vi "ActuationTransform_v6.vi"(8 "1/Actuation Radius":fxp<+,18,0>, 9 "U_thY":fxp<+/-,35,11>, 10 "U_thX":fxp<+/-,35,11>, 11 "U_z":fxp<+/-,35,11>) -> (1 "F_B (Left,B)":fxp<+/-,25,3> format="%.10f", 2 "F_G (Right, G)":fxp<+/-,25,3> format="%.10f", 3 "F_R (Top,R)":fxp<+/-,25,3> format="%.10f")   [LabVIEW 2020, in "FPGA functions.lvlib"]
doc: "Actuation transformation block\n\nFor 3 actuators placed radially symmetrically, translates control effort for gap and tip, tilt into Voltage commands for the electrodes.\n\nv2: Uses lesser number of multiplication blocks!"
uses:
  FPGA functions.lvlib
  <vilib>/Platform/TimedLoop/XDataNode/timing_clust.ctl
  <vilib>/Platform/TimedLoop/XDataNode/nitl_modes.ctl
  <vilib>/Platform/TimedLoop/XDataNode/wakeup.ctl
  <vilib>/rvi/Emulation/niFpgaSctlEmulationGetInTimedLoop.vi
  <vilib>/rvi/Emulation/niFpgaEmulationReportErrorSimple.vi
  <vilib>/rvi/Emulation/niFpgaGetClockAttributes.vi
  <vilib>/rvi/Emulation/niFpgaCriticalErrorInLSC.vi
  <vilib>/Platform/TimedLoop/XDataNode/XDataNode.xnode
  <vilib>/rvi/FXPMathLib/FxpMul/XNode/nifxpmath_Multiplier.xnode
  <vilib>/rvi/FXPMathLib/FxpSub/XNode/nifxpmath_Sub.xnode
  <vilib>/rvi/FXPMathLib/FxpAdd/XNode/nifxpmath_Add.xnode
  <vilib>/rvi/FXPMathLib/sim/FxpSim.dll
  <vilib>/Platform/TimedLoop/XDataNode/XDNodeRunTimeDep.lvlib
panel:
  # "- force (scaled)"
  # "- torque (scaled)"
  # "- torque (scaled)"
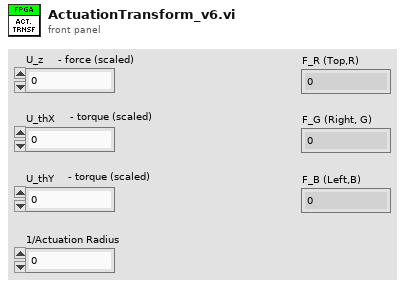
[diagram p1: front panel]
types:
  T1 = typedef "XDNodeRunTimeDep.lvlib/timing_clust.ctl" = cluster{"Expected End [f-1]":u64, "Actual End [f-1]":u64, "Finished Late? [f-1]":bool, "Expected End [i-1]":u64, "Actual End [i-1]":u64, "Finished Late? [i-1]":bool, "Expected Start [i]":u64, "Actual Start [i]":u64, "Expected Start [f]":u64, "Actual Start [f]":u64, "Source Name":string, "Structure Name":string, "Period":i64, "Deadline":i64, "Offset":i64, "Start":i64, "Priority":i32, "Timeout":i32, "Mode":T2, "Wakeup Reason":T3, "Error":errorcluster, "Source Type":string, "Secondary Source Type":string, "Global End Time":u64, "Global Start Time":u64, "Frame Duration":u64, "Iteration Duration":u64, "Assigned CPU":i32, "I/O Scan Engine Mode":u32}
  T2 = typedef "XDNodeRunTimeDep.lvlib/nitl_modes.ctl" = enum32{"No Change", "Process missed periods, maintain original phase", "Discard missed periods, maintain original phase", "Process missed periods, ignore original phase", "Discard missed periods, ignore original phase"}
  T3 = typedef "XDNodeRunTimeDep.lvlib/wakeup.ctl" = enum32{"Normal", "Aborted", "Asynchronous wakeup", "Timing source error", "Timed loop error", "Timeout"}
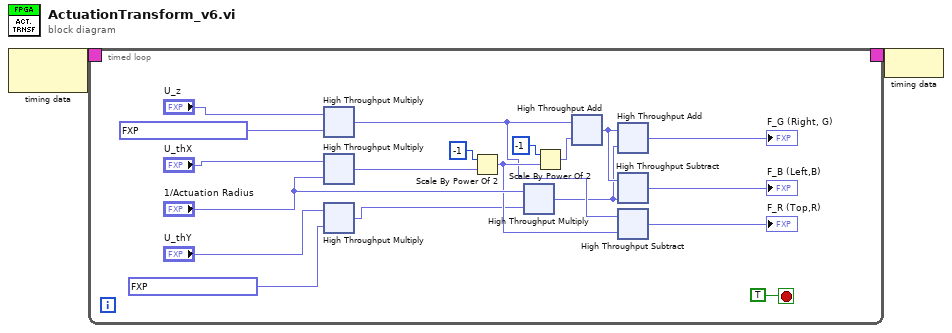
[diagram p0: block diagram]
diagram:
  n1 = node-c288() -> (w2:T1)  [unwired: 1 in]
  n2 = timed-loop {
    timing: w2 -> [_]
    timing-out: [_] -> w1
    stop <- TRUE stop-if-true
    n3 = xnode ("High Throughput Multiply")("x"="U_z", "y"=fxp<+/-,18,0> -0.3333320617675781) -> ("x*y"=w7:fxp<+/-,37,13>)
    n4 = xnode ("High Throughput Multiply")("x"="U_thX", "y"="1/Actuation Radius") -> ("x*y"=w5:fxp<+/-,39,13>)
    n5 = xnode ("High Throughput Multiply")("x"="U_thY", "y"=fxp<+,18,-1> 0.28867530822753906) -> ("x*y"=w6:fxp<+/-,37,13>)
    n6 = Scale By Power Of 2(n=i16 -1, x=w5) -> (x*2^n=w10:fxp<+/-,39,13>)
    n7 = xnode ("High Throughput Multiply")("x"="1/Actuation Radius", "y"=w6) -> ("x*y"=w4:fxp<+/-,37,12>)
    n8 = Scale By Power Of 2(n=i16 -1, x=w10) -> (x*2^n=w8:fxp<+/-,39,13>)
    n9 = xnode ("High Throughput Add")("x"=w7, "y"=w8) -> ("x+y"=w12:fxp<+/-,38,14>)
    n10 = xnode ("High Throughput Add")("x"=w12, "y"=w4) -> ("x+y"=→"F_G (Right, G)":fxp<+/-,25,3>)
    n11 = xnode ("High Throughput Subtract")("x"=w12, "y"=w4) -> ("x-y"=→"F_B (Left,B)":fxp<+/-,25,3>)
    n12 = xnode ("High Throughput Subtract")("x"=w7, "y"=w10) -> ("x-y"=→"F_R (Top,R)":fxp<+/-,25,3>)
  }
  n13 = node-c288(w1) -> ()
